vi "Configure Meas Complete Dest [MP].vi"(8 "error in (no error)":errorcluster, 10 "meas complete dest (None)":i32(ring)=-1 items=["None"=-1, "External"=2, "PXI TRIG0 or VXI TTL0"=111, "PXI TRIG1 or VXI TTL1"=112, "PXI TRIG2 or VXI TTL2"=113, "PXI TRIG3 or VXI TTL3"=114, "PXI TRIG4 or VXI TTL4"=115, "PXI TRIG5 or VXI TTL5"=116, "PXI TRIG6 or VXI TTL6"=117, "PXI TRIG7 or VXI TTL7"=118, "ECL0"=119, "ECL1"=120, "PXI Star"=131, "RTSI 0"=140, "RTSI 1"=141, "RTSI 2"=142, "RTSI 3"=143, "RTSI 4"=144, "RTSI 5"=145, "RTSI 6"=146], 11 "CS++DMM in":refnum<class "CS++DMM.lvclass">) -> (0 "error out":errorcluster, 3 "CS++DMM out":refnum<class "CS++DMM.lvclass">)   [LabVIEW 2013, in "CS++DMM.lvlib" / "CS++DMM.lvclass"]
doc: "This VI configures the destination of the measurement-complete signal. This signal is commonly referred to as Voltmeter Complete.\n\nNote:\n\n(1) This VI is part of the IviDmmMultiPoint [MP] extension group."
uses:
  CS++DMM.lvclass
  CSPP_Core/Classes/CS++ProcessVariables/ProcessVariable/PV.lvclass
  CSPP_Core/Classes/CS++ProcessVariables/ProcessVariable/PV.lvclass/PV.ctl
  CS++DMM.lvclass/CS++DMM.ctl
  CSPP_Core/Classes/CS++ProcessVariables/PVConnection/PVConnection.lvclass
  CSPP_Core/Classes/CS++ProcessVariables/ProcessVariable/Write Data.vi
  CSPP_Core/Classes/CS++ProcessVariables/ProcessVariable/Write Timestamp.vi
  CSPP_Core/Classes/CS++ProcessVariables/ProcessVariable/Write Quality.vi
  CSPP_Core/Classes/CS++ProcessVariables/ProcessVariable/Write status.vi
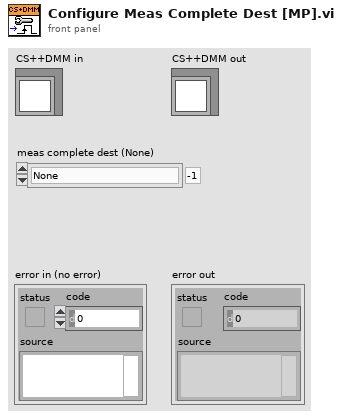
[diagram p1: front panel]
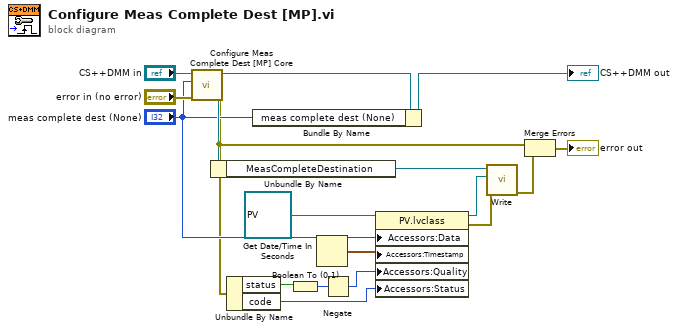
[diagram p0: block diagram]
diagram:
  n1 = call-dynamic "Configure Meas Complete Dest [MP] Core.vi"("error in (no error)"="error in (no error)", "meas complete dest (None)"="meas complete dest (None)", "CS++DMM in"="CS++DMM in") -> ("error out"=w3:errorcluster, "CS++DMM out"=w6:refnum<class "CS++DMM.lvclass">)  [unwired: 7 in]
  n2 = Unbundle By Name(w6) -> ("MeasCompleteDestination"=w5:refnum<class "PVConnection.lvclass">)
  n3 = Unbundle By Name(w3) -> ("status"=w13:bool, "code"=w10:i32)
  n4 = Bundle By Name(cluster=w6, "meas complete dest (None)"="meas complete dest (None)") -> (→"CS++DMM out":refnum<class "CS++DMM.lvclass">)
  n5 = Boolean To (0,1)(Boolean=w13) -> (0, 1=w12:i16)
  n6 = Get Date/Time In Seconds() -> (seconds since 1Jan1904=w9:timestamp)
  n7 = Negate(x=w12) -> (-x=w11:i16)
  n8 = property class="PV.lvclass"(reference=refnum<class "PV.lvclass"> refnum ("CS++ProcessVariables.lvlib:PV.lvclass"), "Accessors:Data"="meas complete dest (None)", "Accessors:Timestamp"=w9, "Accessors:Quality"=w11, "Accessors:Status"=w10) -> (reference out=w7:refnum<class "PV.lvclass">, error out=w8:errorcluster)  [unwired: 1 in]
  n9 = call-dynamic "Write.vi"("error in (no error)"=w8, "PV"=w7, "PVConnection in"=w5) -> ("error out"=w2:errorcluster)  [unwired: 7 in, 1 out]
  n10 = Merge Errors(w3, w2) -> (→"error out":errorcluster)
